vi "sendconfiguration.vi"(8 "error in (no error)":errorcluster, 10 "pData":u8[](array[numeric]) format="%.0x", 11 "hObject":i32) -> (0 "error out":errorcluster, 3 "hObject Out":i32)   [LabVIEW 2018]
doc: "this vi sends the configuration from the device\n\n12/21/2010 1.0.0 jyg\n- initial release"
uses:
  icsneo40.dll
panel:
  in  "pINumBytes":i32
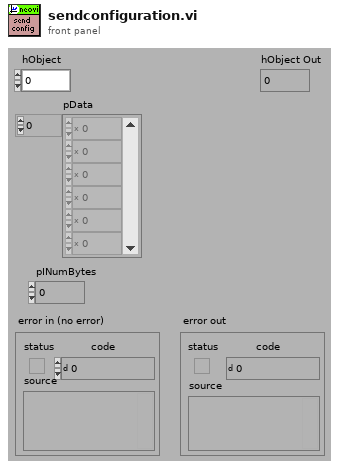
[diagram p1: front panel]
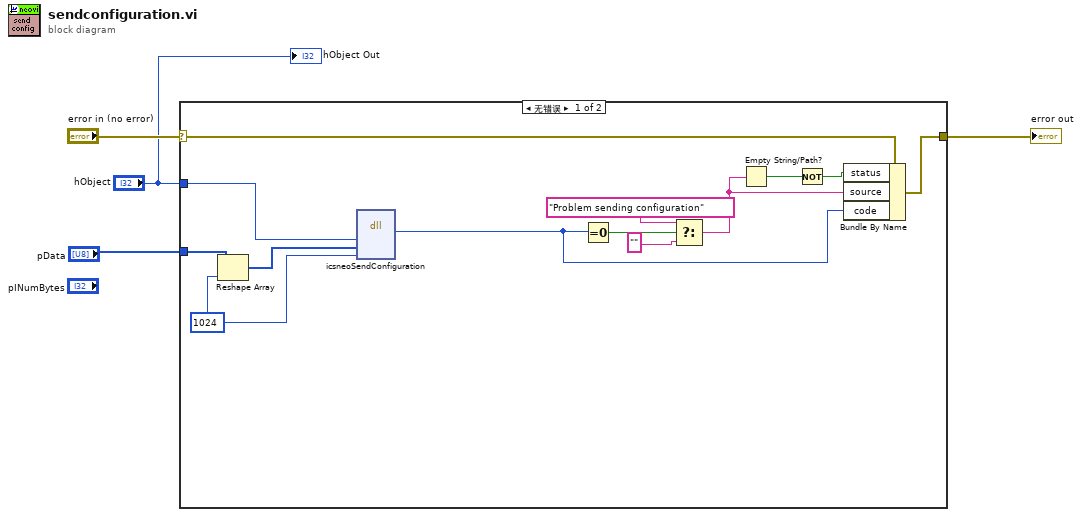
[diagram p0: block diagram]
diagram:
  n1 = case shown="无错误" "error in (no error)" {
    selector: "error in (no error)" -> [w13 w18]
    tunnel: "hObject" -> [w8 _]
    tunnel: [w14 w18] -> w4
    tunnel: "pData" -> [w7 _]
    frame No Error {
      w6 = 1024 ("1NumBytes")
      n2 = Reshape Array(w7, w6) -> (w5:u8[])
      n3 = dll-call lib="icsneo40.dll" fn="icsneoSendConfiguration"("hObject"=w8, "pData"=w5, "1NumBytes"=w6) -> ("return type"=w12:i32)  [unwired: 6 in, 2 out]
      n4 = Equal To 0?(x=w12) -> (x = 0?=w11:bool)
      n5 = Select(t="Problem sending configuration", s=w11, f="") -> (s? t:f=w10:string)
      n6 = Empty String/Path?(string/path=w10) -> (empty?=w16:bool)
      n7 = Not(x=w16) -> (.not. x?=w15:bool)
      n8 = Bundle By Name(cluster=w13, "status"=w15, "source"=w10, "code"=w12) -> (w14:errorcluster)
    }
    frame Error {
    }
  }
  "error out" <- w4
  "hObject Out" <- "hObject"
